vi "CreateTask.vi"(8 "error in":errorcluster, 11 "MainFGV_data":T1) -> (0 "error out":errorcluster, 3 "MainFGV_data out":T1)   [LabVIEW 2016]
uses:
  MainFGV_data.ctl
  config_board.ctl
  <vilib>/DAQmx/create/channels.llb/DAQmx Create Channel (AI-Acceleration-Accelerometer).vi
  <resource>/objmgr/daqmx.rc
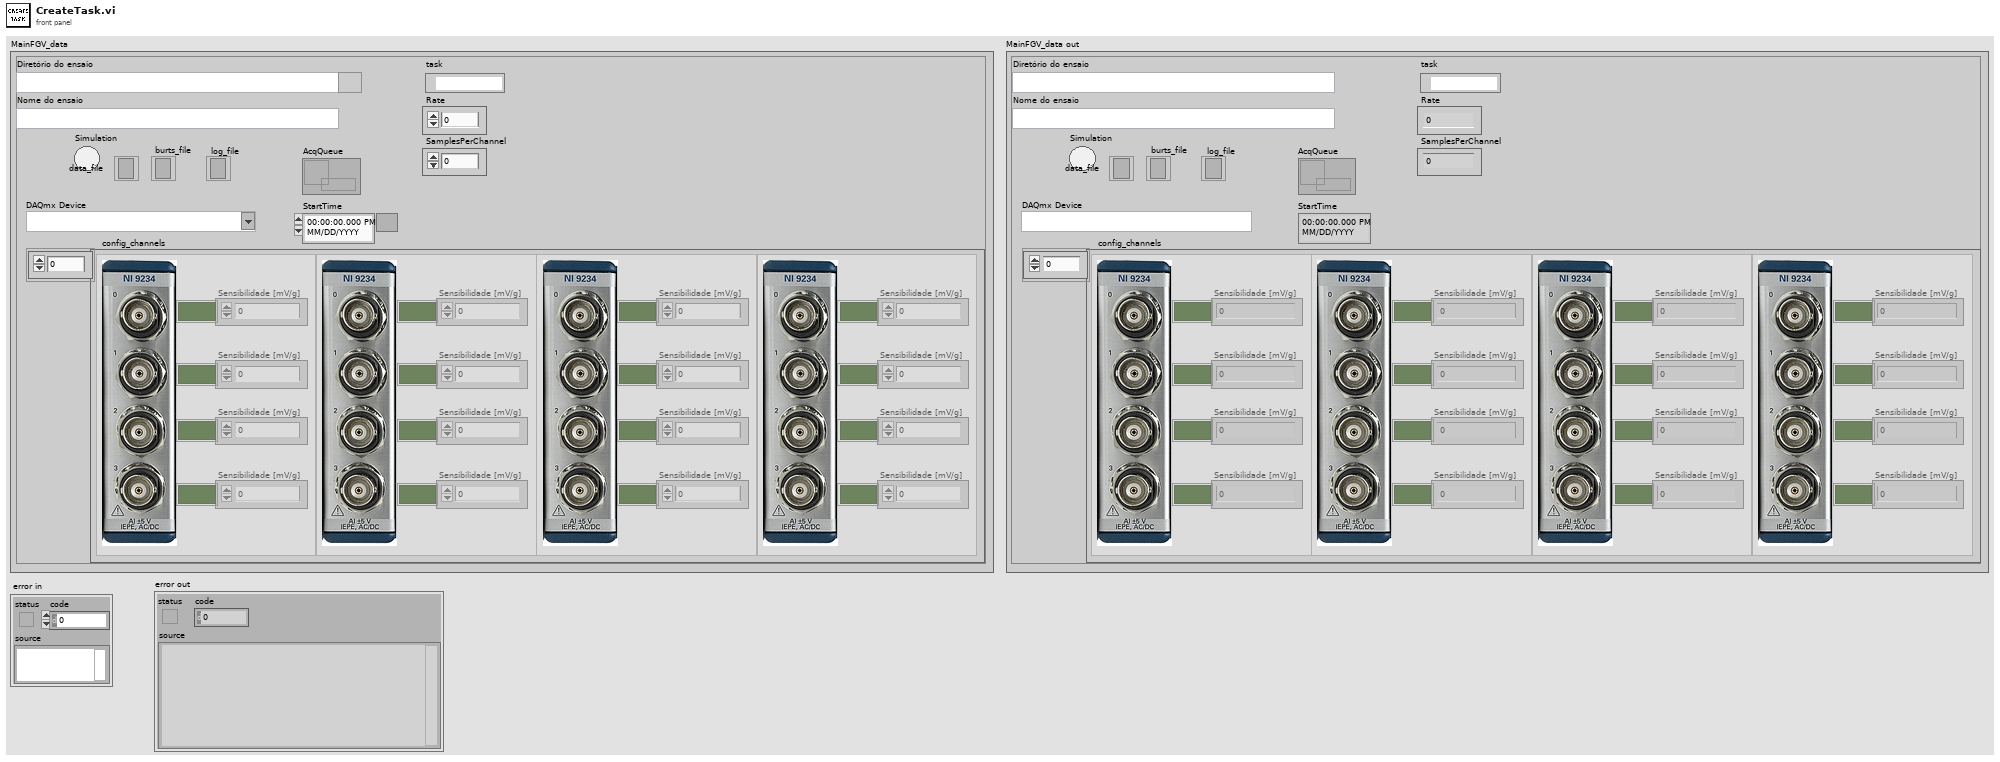
[diagram p1: front panel]
types:
  T1 = typedef "MainFGV_data.ctl" = cluster{"TestDir":path, "TestName":string, "Simulation":bool, "task":refnum<k21>, "data_file":refnum<file>, "burts_file":refnum<file>, "log_file":refnum<file>, "Rate":dbl, "SamplesPerChannel":dbl, "AcqQueue":refnum<queue>, "StartTime":timestamp, "config_channels":T2[], "DAQmx Device":tag}
  T2 = typedef "config_board.ctl" = cluster{"Sens0":dbl, "Active0":bool, "Sens1":dbl, "Active1":bool, "Sens2":dbl, "Active2":bool, "Sens3":dbl, "Active3":bool}
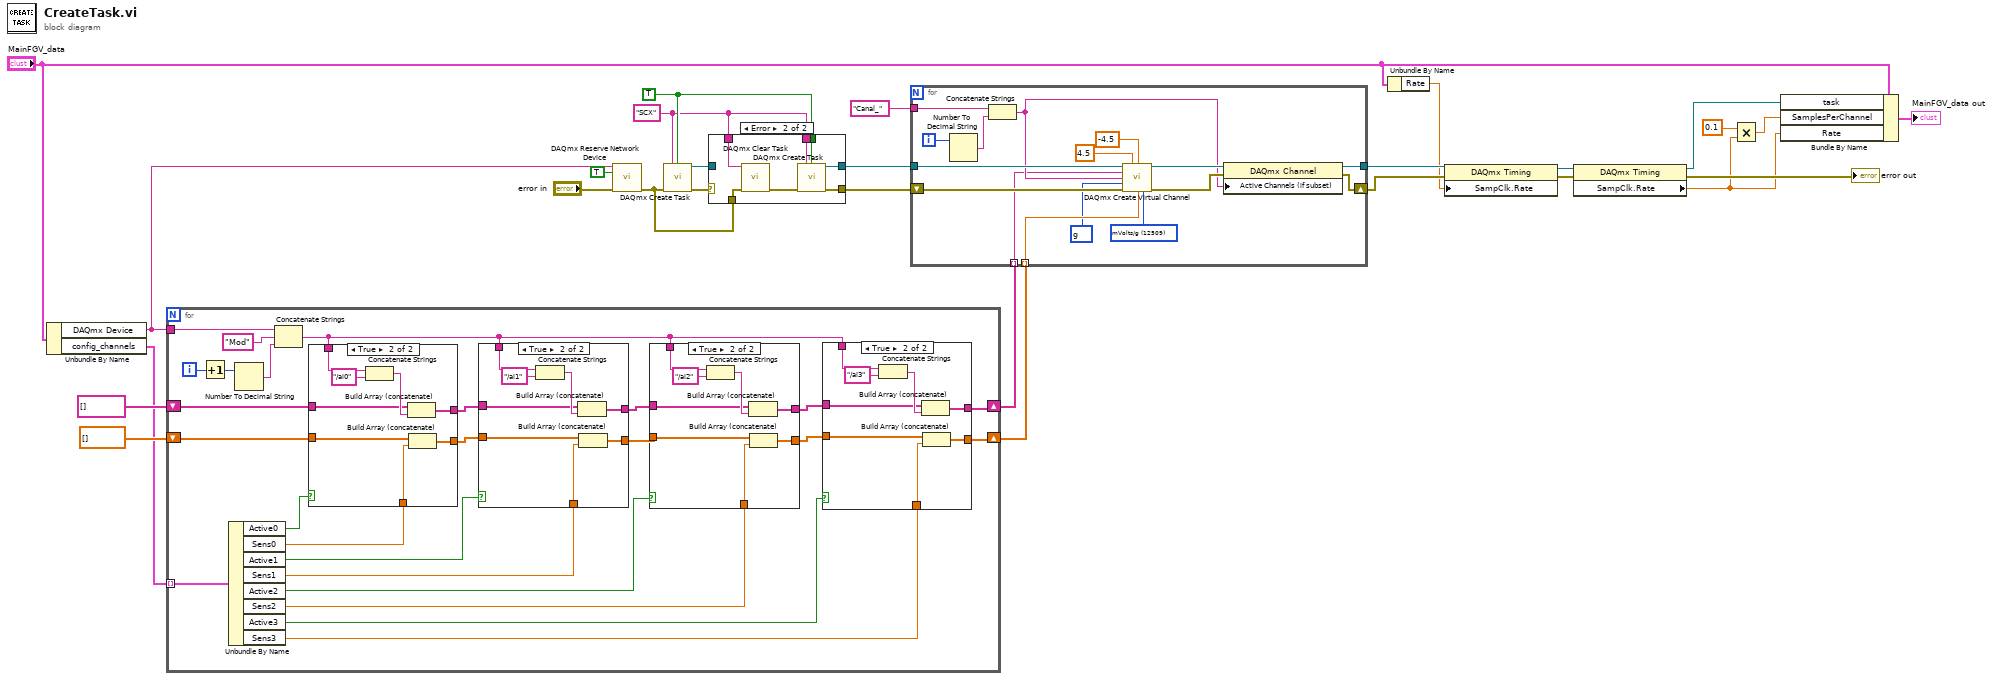
[diagram p0: block diagram]
diagram:
  w25 = TRUE ("auto cleanup")
  w24 = "SCX" ("new task name")
  n1 = Unbundle By Name("MainFGV_data") -> ("DAQmx Device"=w4:tag, "config_channels"=w14:T2[])
  n2 = for {
    tunnel: w14 -> [w53] mode=indexing
    tunnel: w4 -> [w51]
    shift-right: [w30] -> w18
    shift-left: string[] [] -> [w46]
    shift-right: [w29] -> w17
    shift-left: dbl[] [] ("Sensibilidades [mV/g]") -> [w45]
    i -> [w52]
    n3 = Increment(x=w52) -> (x+1=w49:i32)
    n4 = Unbundle By Name(w53) -> ("Active0"=w47:bool, "Sens0"=w44:dbl, "Active1"=w34:bool, "Sens1"=w37:dbl, "Active2"=w33:bool, "Sens2"=w36:dbl, "Active3"=w32:bool, "Sens3"=w35:dbl)
    n5 = Number To Decimal String(number=w49) -> (decimal integer string=w48:string)  [unwired: 1 in]
    n6 = Concatenate Strings(w51, "Mod" ("string"), w48) -> (w41:string)
    n7 = case shown="True" w47 {
      tunnel: w41 -> [_ w93]
      tunnel: w46 -> [w85 w90]
      tunnel: w45 -> [w84 w89]
      tunnel: w44 -> [_ w86]
      tunnel: [w85 w88] -> w43
      tunnel: [w84 w87] -> w31
      frame False {
      }
      frame True {
        n8 = Concatenate Strings(w93, "/ai0" ("string")) -> (w91:string)
        n9 = Build Array (concatenate)(w90, w91) -> (w88:string[])
        n10 = Build Array (concatenate)(w89, w86) -> (w87:dbl[])
      }
    }
    n11 = case shown="True" w34 {
      tunnel: w41 -> [_ w83]
      tunnel: w43 -> [w75 w80]
      tunnel: w31 -> [w74 w79]
      tunnel: w37 -> [_ w76]
      tunnel: [w75 w78] -> w42
      tunnel: [w74 w77] -> w38
      frame False {
      }
      frame True {
        n12 = Concatenate Strings(w83, "/ai1" ("string")) -> (w81:string)
        n13 = Build Array (concatenate)(w80, w81) -> (w78:string[])
        n14 = Build Array (concatenate)(w79, w76) -> (w77:dbl[])
      }
    }
    n15 = case shown="True" w33 {
      tunnel: w41 -> [_ w73]
      tunnel: w42 -> [w65 w70]
      tunnel: w38 -> [w64 w69]
      tunnel: w36 -> [_ w66]
      tunnel: [w65 w68] -> w40
      tunnel: [w64 w67] -> w39
      frame False {
      }
      frame True {
        n16 = Concatenate Strings(w73, "/ai2" ("string")) -> (w71:string)
        n17 = Build Array (concatenate)(w70, w71) -> (w68:string[])
        n18 = Build Array (concatenate)(w69, w66) -> (w67:dbl[])
      }
    }
    n19 = case shown="True" w32 {
      tunnel: w41 -> [_ w63]
      tunnel: w40 -> [w55 w60]
      tunnel: w39 -> [w54 w59]
      tunnel: w35 -> [_ w56]
      tunnel: [w55 w58] -> w30
      tunnel: [w54 w57] -> w29
      frame False {
      }
      frame True {
        n20 = Concatenate Strings(w63, "/ai3" ("string")) -> (w61:string)
        n21 = Build Array (concatenate)(w60, w61) -> (w58:string[])
        n22 = Build Array (concatenate)(w59, w56) -> (w57:dbl[])
      }
    }
  }
  n23 = call <vilib>:"DAQmx Reserve Network Device.vi"("device in"=w4, "override reservation?"=TRUE, "error in"="error in") -> ("error out"=w1:errorcluster)  [unwired: 11 in, 1 out]
  n24 = call <vilib>:"DAQmx Create Task.vi"("new task name"=w24, "auto cleanup"=w25, "error in"=w1) -> ("task out"=w26:refnum<k21>, "error out"=w27:errorcluster)  [unwired: 11 in]
  n25 = case shown="Error" w27 {
    selector: w27 -> [w94 _]
    tunnel: w26 -> [w95 _]
    tunnel: [w95 w97] -> w12
    tunnel: w1 -> [_ w102]
    tunnel: [w94 w100] -> w13
    tunnel: w25 -> [_ w99]
    tunnel: w24 -> [_ w98]
    tunnel: w24 -> [_ w96]
    frame No Error {
    }
    frame Error {
      n26 = call <vilib>:"DAQmx Clear Task.vi"("task in"=w96, "error in"=w102) -> ("error out"=w101:errorcluster)  [unwired: 13 in]
      n27 = call <vilib>:"DAQmx Create Task.vi"("new task name"=w98, "auto cleanup"=w99, "error in"=w101) -> ("task out"=w97:refnum<k21>, "error out"=w100:errorcluster)  [unwired: 11 in]
    }
  }
  n28 = for {
    tunnel: w12 -> [w118]
    shift-right: [w109] -> w23
    shift-left: w13 -> [w117]
    tunnel: [w111] -> w21
    tunnel: w17 -> [w116] mode=indexing
    tunnel: "Canal_" ("new task name") -> [w113]
    tunnel: w18 -> [w107] mode=indexing
    i -> [w115]
    w103 = 10186 items=["g"=10186, "m/s^2"=12470, "in/s^2"=12471, "From Custom Scale"=10065] ("units")
    w104 = 12509 items=["mVolts/g"=12509, "Volts/g"=12510] ("sensitivity units")
    n29 = Number To Decimal String(number=w115) -> (decimal integer string=w114:string)  [unwired: 1 in]
    n30 = Concatenate Strings(w113, w114) -> (w108:string)
    n31 = call-poly <vilib>:"DAQmx Create Virtual Channel.vi"("task in"=w118, "maximum value"=4.5, "minimum value"=-4.5, "physical channels"=w107, "name to assign"=w108, "units"=w103, "error in"=w117, "sensitivity"=w116, "sensitivity units"=w104) -> ("task out"=w112:refnum<k21>, "error out"=w110:errorcluster)  [unwired: 5 in]
    n32 = property class="DAQmx Channel"(reference=w112, error in=w110, "Active Channels (if subset)"=w108) -> (reference out=w111:refnum<k21>, error out=w109:errorcluster)
  }
  n33 = Unbundle By Name("MainFGV_data") -> ("Rate"=w5:dbl)
  n34 = property class="DAQmx Timing"(reference=w21, error in=w23, "SampClk.Rate"=w5) -> (reference out=w16:refnum<k21>, error out=w15:errorcluster)
  n35 = property class="DAQmx Timing"(reference=w16, error in=w15) -> (reference out=w10:refnum<k21>, error out=→"error out":errorcluster, "SampClk.Rate"=w7:dbl)
  n36 = Multiply(x=0.1 ("y"), y=w7) -> (x*y=w8:dbl)
  n37 = Bundle By Name(cluster="MainFGV_data", "task"=w10, "SamplesPerChannel"=w8, "Rate"=w7) -> (→"MainFGV_data out":T1)
